vi "BRig_RT_panel_Laser1_v0,902.vi"(7 "input_setValues":bool, 9 "input_dataExp":u16[](array[numeric]), 11 "input_dataLC":u16[](array[numeric])) -> (1 "output_dataExp":u16[](array[numeric]), 3 "output_dataLC":u16[](array[numeric]))   [LabVIEW 2014]
panel:
  out "LaserPulseTrain":cluster{u16[], u16[]}(graph)
  in  "LED_baseline":bool
  in  "Laser_power_step":dbl
  in  "Laser_power_max":dbl
  in  "Laser_power_min":dbl
  in  "Laser_Tshutter":u16=2
  in  "Laser_Freq":u16=10
  in  "Laser_Tpeak":u16=2
  in  "Laser_T":u16
  in  "LC_Sel_PostR_Count":u16
  in  "LC_Sel_PostR_Probability":u16
  in  "LC_Sel_PostR_Block":u16(slide) max=2 step=1 scale=0.0..2.0
  in  "LC_Sel_PostR_OnOff":bool
  in  "LC_Sel_PostR_Tdelay":u16
  in  "LC_Cue_PostR_Count":u16
  in  "LC_Cue_PostR_delayOpt":bool
  in  "LC_Cue_PostR_Probability":u16
  in  "LC_Cue_PostR_Block":u16(slide) max=2 step=1 scale=0.0..2.0
  in  "LC_Cue_PostR_OnOff":bool
  in  "LC_Cue_PostR_Tdelay":u16
  in  "LC_ENL_PostR_delayOpt":bool
  in  "LC_ENL_PostR_Count":u16
  in  "LC_ENL_PostR_Probability":u16 max=100 step=1
  in  "LC_ENL_PostR_Block":u16(slide) max=2 step=1 scale=0.0..2.0
  in  "LC_ENL_PostR_OnOff":bool
  in  "LC_ENL_PostR_Tdelay":u16
  in  "LC_Sel_PreR_Count":u16
  in  "LC_Sel_First_Count":u16
  in  "LC_Sel_PreR_Probability":u16
  in  "LC_Sel_PreR_Block":u16(slide) max=2 step=1 scale=0.0..2.0
  in  "LC_Sel_PreR_OnOff":bool
  in  "LC_Sel_First_Probability":u16
  in  "LC_Sel_First_Block":u16(slide) max=2 step=1 scale=0.0..2.0
  in  "LC_Sel_First_OnOff":bool
  in  "LC_Sel_PreR_Tdelay":u16
  in  "LC_Sel_First_Tdelay":u16
  in  "LC_Cue_PreR_Count":u16
  in  "LC_Cue_First_Count":u16
  in  "LC_Cue_PreR_delayOpt":bool
  in  "LC_ENL_PreR_delayOpt":bool
  in  "LC_ENL_PreR_Count":u16
  in  "LC_ENL_First_Count":u16
  in  "LC_Cue_First_delayOpt":bool
  in  "LC_ENL_First_delayOpt":bool
  in  "LC_Wrong_Probability":u16
  in  "LC_Wrong_Trial":u16(slide) max=2 step=1 scale=0.0..2.0
  in  "LC_Wrong_Block":u16(slide) max=2 step=1 scale=0.0..2.0
  in  "LC_Wrong_OnOff":bool
  in  "LC_Reward_Probability":u16
  in  "LC_Reward_Trial":u16(slide) max=2 step=1 scale=0.0..2.0
  in  "LC_Reward_Block":u16(slide) max=2 step=1 scale=0.0..2.0
  in  "LC_Reward_OnOff":bool
  in  "LC_Cue_PreR_Probability":u16
  in  "LC_Cue_PreR_Block":u16(slide) max=2 step=1 scale=0.0..2.0
  in  "LC_Cue_PreR_OnOff":bool
  in  "LC_Cue_First_Probability":u16
  in  "LC_Cue_First_Block":u16(slide) max=2 step=1 scale=0.0..2.0
  in  "LC_Cue_First_OnOff":bool
  in  "LC_ENL_PreR_Probability":u16 max=100 step=1
  in  "LC_ENL_PreR_Block":u16(slide) max=2 step=1 scale=0.0..2.0
  in  "LC_ENL_PreR_OnOff":bool
  in  "LC_ENL_First_Probability":u16 max=100 step=1
  in  "LC_ENL_First_Block":u16(slide) max=2 step=1 scale=0.0..2.0
  in  "LC_Wrong_Tdelay":u16
  in  "LC_Cue_PreR_Tdelay":u16
  in  "LC_ENL_PreR_Tdelay":u16
  in  "LC_Reward_Tdelay":u16
  in  "LC_Cue_First_Tdelay":u16
  in  "LC_ENL_First_Tdelay":u16
  in  "LC_ENL_First_OnOff":bool
  # "Laser1 Control\n                               On/Off      Block        Probability [%]   Delay [ms]                              Count"
  # "Enforced\nNonLick"
  # "from end"
  # "First\nTrial"
  # "from start"
  # "from end"
  # "PreReward\nTrials"
  # "from start"
  # "from end"
  # "PostReward\nTrials"
  # "from start"
  # "Cue"
  # "from end"
  # "First\nTrial"
  # "from start"
  # "from end"
  # "PreReward\nTrials"
  # "from start"
  # "from end"
  # "PreReward\nTrials"
  # "from start"
  # "Selection"
  # "from start"
  # "First\nTrial"
  # "from start"
  # "PreReward\nTrials"
  # "from start"
  # "PostReward\nTrials"
  # "Laser1 Parameters"
  # "Laser1 Response\n           On/Off      Block           Trial     Probability %  Delay [ms]"
  # "Frequency\n[Hz]"
  # "Selection\nReward"
  # "Timing [ms]\n Duration     Peak Width   Shutter"
  # "Selection\nWrong"
  # "Laser Power [V]\nMin          Max              Step"
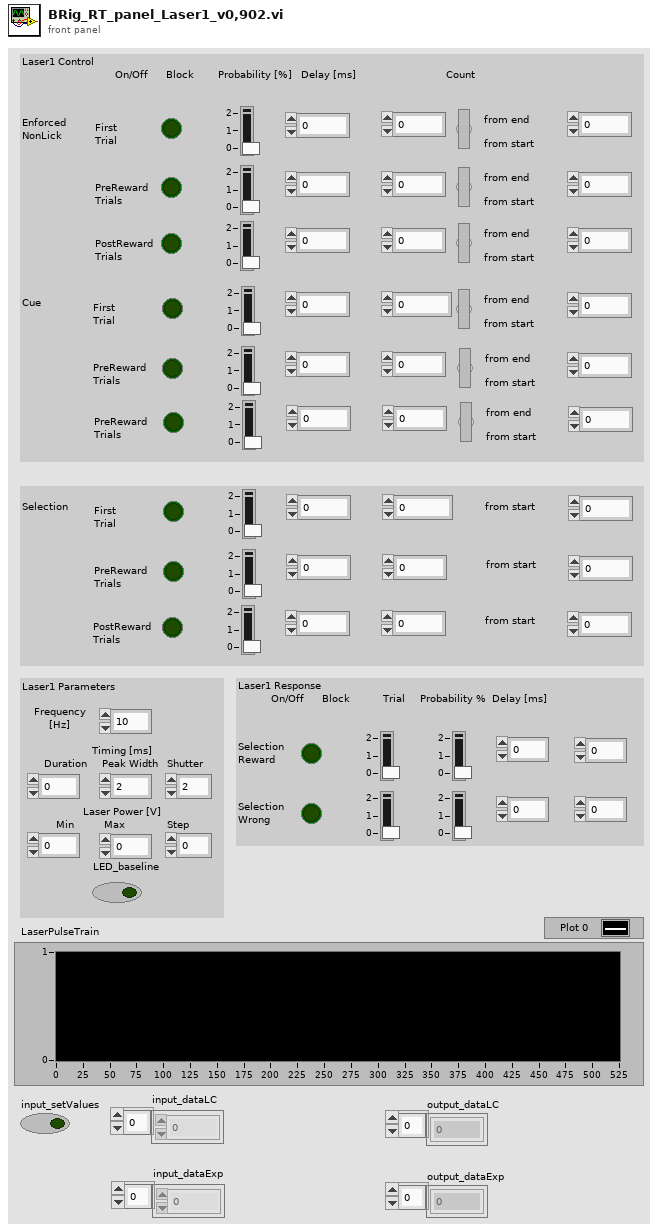
[diagram p1: front panel]
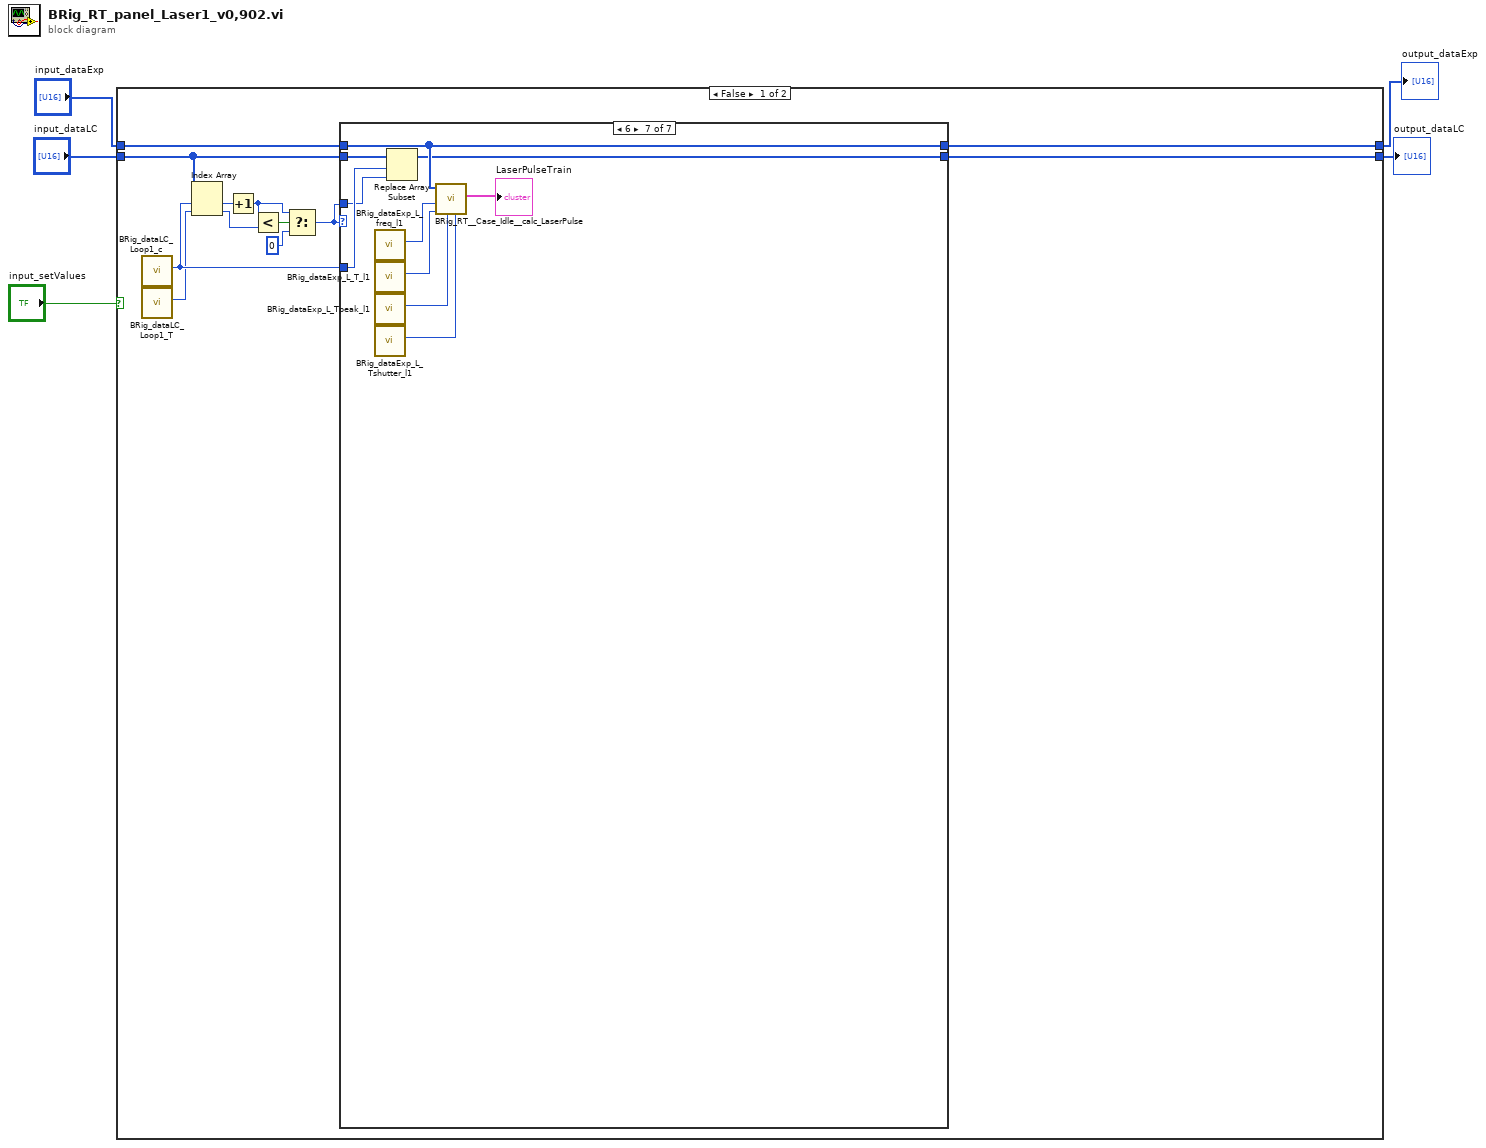
[diagram p0: block diagram]
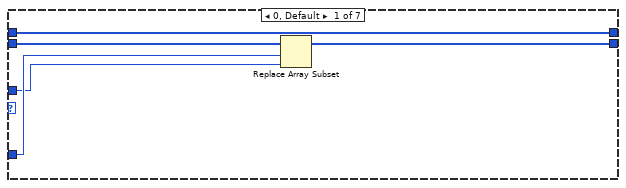
[diagram p2: hidden frame]
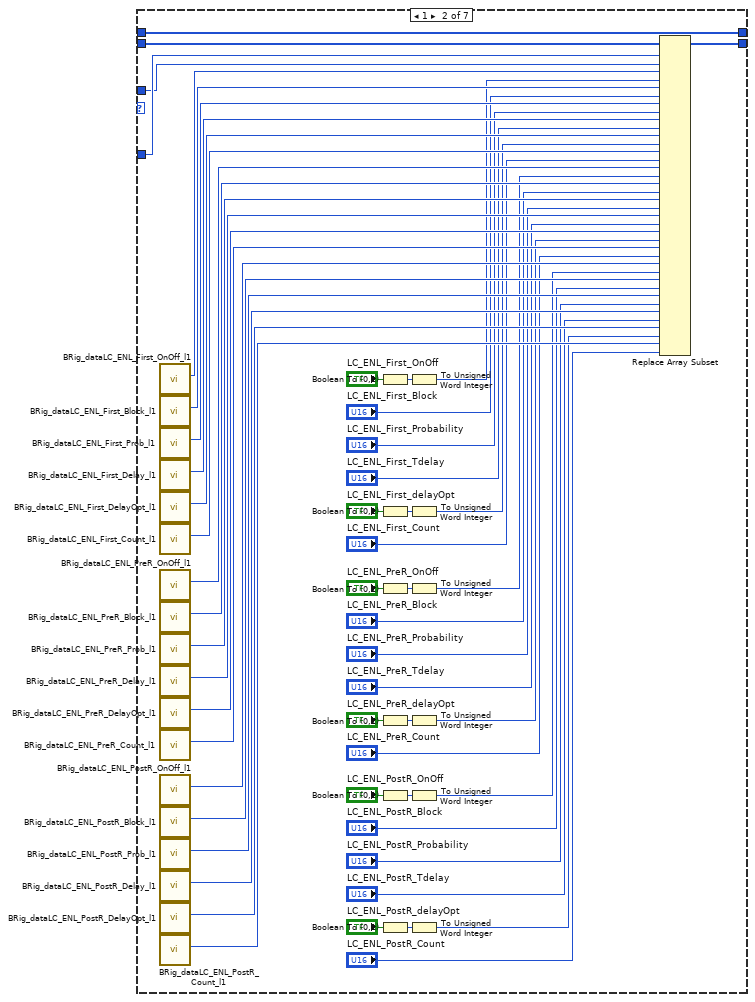
[diagram p3: hidden frame]
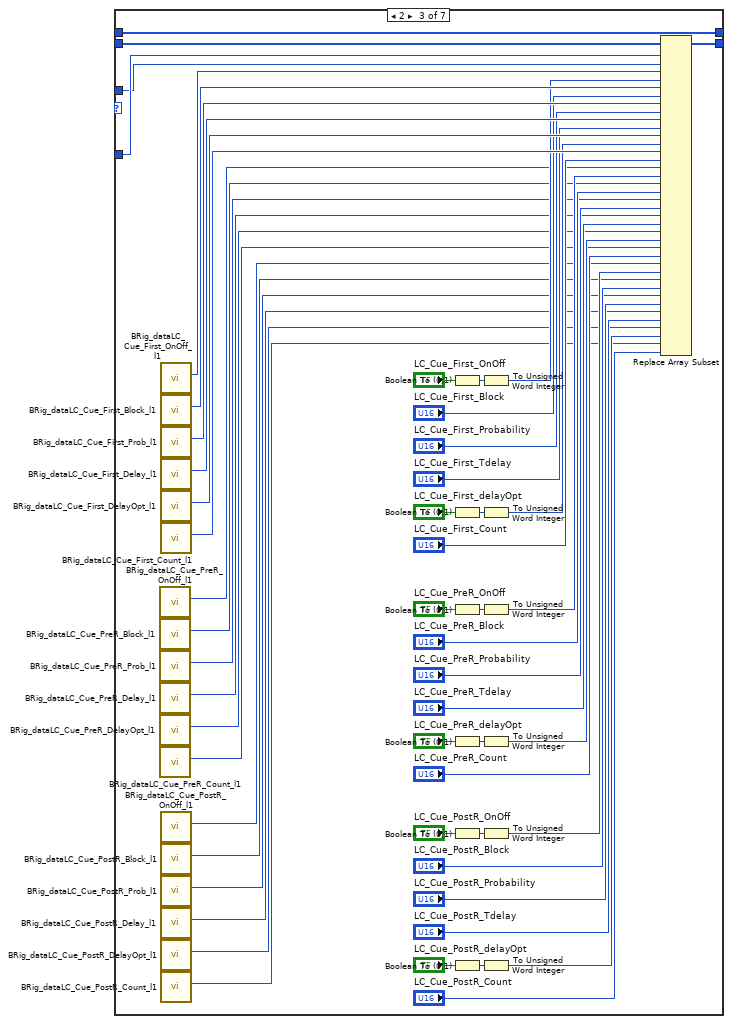
[diagram p4: hidden frame]
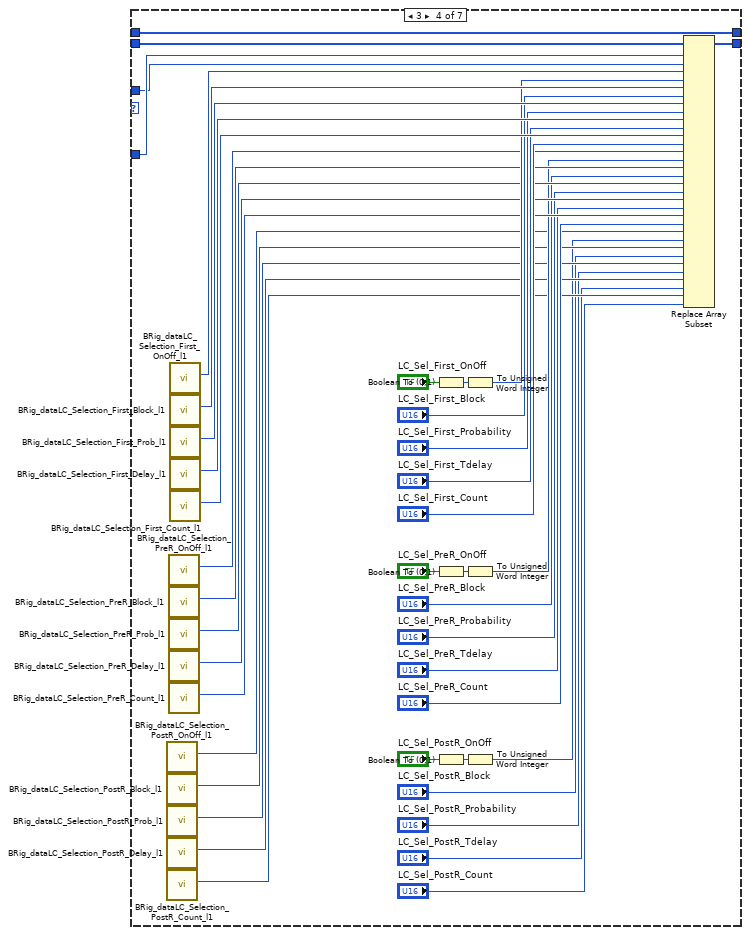
[diagram p5: hidden frame]
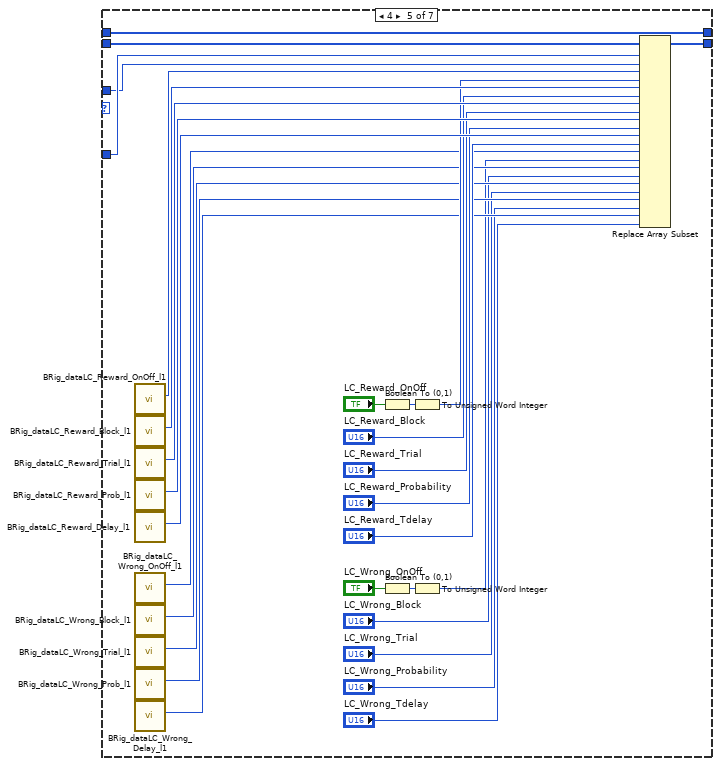
[diagram p6: hidden frame]
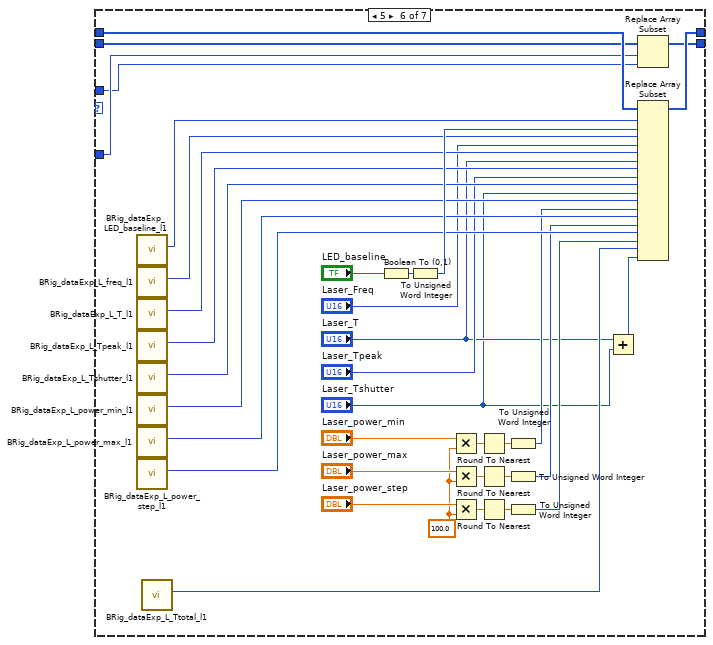
[diagram p7: hidden frame]
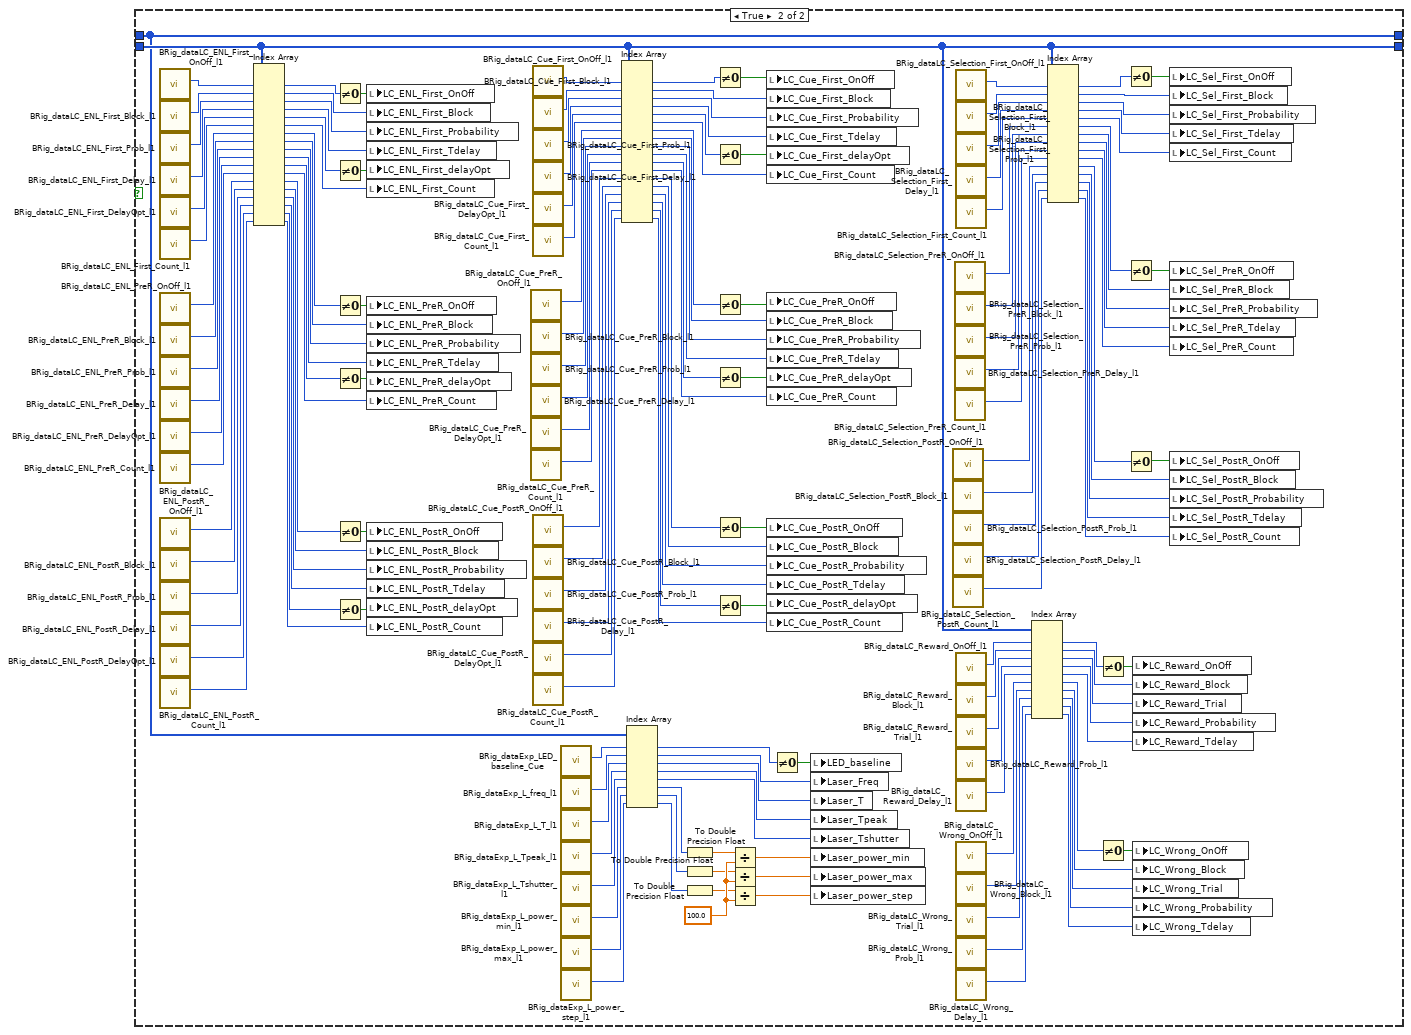
[diagram p8: hidden frame]
diagram:
  n1 = case shown="False" "input_setValues" {
    tunnel: "input_dataLC" -> [w17 w282]
    tunnel: [w11 w282] -> w4
    tunnel: "input_dataExp" -> [w7 w245]
    tunnel: [w6 w245] -> w1
    frame False {
      n2 = call "BRig_dataLC_Loop1_c.vi"() -> ("output_Loop1_c"=w10:i32)  [unwired: 11 in]
      n3 = call "BRig_dataLC_Loop1_T.vi"() -> ("output_Loop1_T"=w9:i32)  [unwired: 11 in]
      n4 = Index Array(array=w17, index #1=w10, index #2=w9) -> (element #1=w16:u16, element #2=w15:u16)
      n5 = Increment(x=w16) -> (x+1=w12:u16)
      n6 = Less?(x=w12, y=w15) -> (x < y?=w14:bool)
      n7 = Select(t=w12, s=w14, f=u16 0) -> (s? t:f=w8:u16)
      n8 = case shown="6" w8 {
        tunnel: w17 -> [w22 w75 w128 w169 w198 w203 w242]
        tunnel: w10 -> [w20 w25 w90 w131 w172 w201 w240]
        tunnel: w8 -> [w19 w24 w89 w130 w171 w200 w239]
        tunnel: [w21 w68 w127 w168 w197 w202 w241] -> w11
        tunnel: w7 -> [w18 w23 w76 w129 w170 w205 w244]
        tunnel: [w18 w23 w76 w129 w170 w204 w244] -> w6
        frame 0, Default {
          n9 = Replace Array Subset(array=w22, new element=w19, index=w20) -> (w21:u16[])
        }
        frame 1 {
          n10 = call "BRig_dataLC_ENL_First_OnOff_l1.vi"() -> ("output_ENL_First_OnOff"=w74:i32)  [unwired: 11 in]
          n11 = call "BRig_dataLC_ENL_First_Block_l1.vi"() -> ("output_ENL_First_Block"=w73:i32)  [unwired: 11 in]
          n12 = call "BRig_dataLC_ENL_First_Prob_l1.vi"() -> ("output_ENL_First_Prob"=w72:i32)  [unwired: 11 in]
          n13 = call "BRig_dataLC_ENL_First_Delay_l1.vi"() -> ("output_ENL_First_Delay"=w71:i32)  [unwired: 11 in]
          n14 = call "BRig_dataLC_ENL_First_DelayOpt_l1.vi"() -> ("output_ENL_First_DelayOpt"=w70:i32)  [unwired: 11 in]
          n15 = call "BRig_dataLC_ENL_First_Count_l1.vi"() -> ("output_ENL_First_Count"=w69:i32)  [unwired: 11 in]
          n16 = call "BRig_dataLC_ENL_PreR_OnOff_l1.vi"() -> ("output_ENL_PreR_OnOff"=w67:i32)  [unwired: 11 in]
          n17 = call "BRig_dataLC_ENL_PreR_Block_l1.vi"() -> ("output_ENL_PreR_Block"=w66:i32)  [unwired: 11 in]
          n18 = call "BRig_dataLC_ENL_PreR_Prob_l1.vi"() -> ("output_ENL_PreR_Prob"=w65:i32)  [unwired: 11 in]
          n19 = call "BRig_dataLC_ENL_PreR_Delay_l1.vi"() -> ("output_ENL_PreR_Delay"=w64:i32)  [unwired: 11 in]
          n20 = call "BRig_dataLC_ENL_PreR_DelayOpt_l1.vi"() -> ("output_ENL_PreR_DelayOpt"=w63:i32)  [unwired: 11 in]
          n21 = call "BRig_dataLC_ENL_PreR_Count_l1.vi"() -> ("output_ENL_PreR_Count"=w62:i32)  [unwired: 11 in]
          n22 = call "BRig_dataLC_ENL_PostR_OnOff_l1.vi"() -> ("output_ENL_PostR_OnOff"=w61:i32)  [unwired: 11 in]
          n23 = call "BRig_dataLC_ENL_PostR_Block_l1.vi"() -> ("output_ENL_PostR_Block"=w60:i32)  [unwired: 11 in]
          n24 = call "BRig_dataLC_ENL_PostR_Prob_l1.vi"() -> ("output_ENL_PostR_Prob"=w59:i32)  [unwired: 11 in]
          n25 = call "BRig_dataLC_ENL_PostR_Delay_l1.vi"() -> ("output_ENL_PostR_Delay"=w58:i32)  [unwired: 11 in]
          n26 = call "BRig_dataLC_ENL_PostR_DelayOpt_l1.vi"() -> ("output_ENL_PostR_DelayOpt"=w57:i32)  [unwired: 11 in]
          n27 = call "BRig_dataLC_ENL_PostR_Count_l1.vi"() -> ("output_ENL_PostR_Count"=w56:i32)  [unwired: 11 in]
          n28 = Boolean To (0,1)(Boolean="LC_ENL_First_OnOff") -> (0, 1=w54:i16)
          n29 = Boolean To (0,1)(Boolean="LC_ENL_First_delayOpt") -> (0, 1=w53:i16)
          n30 = Boolean To (0,1)(Boolean="LC_ENL_PreR_OnOff") -> (0, 1=w51:i16)
          n31 = Boolean To (0,1)(Boolean="LC_ENL_PreR_delayOpt") -> (0, 1=w49:i16)
          n32 = Boolean To (0,1)(Boolean="LC_ENL_PostR_OnOff") -> (0, 1=w47:i16)
          n33 = Boolean To (0,1)(Boolean="LC_ENL_PostR_delayOpt") -> (0, 1=w45:i16)
          n34 = To Unsigned Word Integer(number=w54) -> (unsigned 16bit integer=w43:u16)
          n35 = To Unsigned Word Integer(number=w53) -> (unsigned 16bit integer=w39:u16)
          n36 = To Unsigned Word Integer(number=w51) -> (unsigned 16bit integer=w37:u16)
          n37 = To Unsigned Word Integer(number=w49) -> (unsigned 16bit integer=w33:u16)
          n38 = To Unsigned Word Integer(number=w47) -> (unsigned 16bit integer=w31:u16)
          n39 = To Unsigned Word Integer(number=w45) -> (unsigned 16bit integer=w27:u16)
          n40 = Replace Array Subset(array=w75, new element #1=w24, index #1=w25, new element #2=w43, index #2=w74, new element #3="LC_ENL_First_Block", index #3=w73, new element #4="LC_ENL_First_Probability", index #4=w72, new element #5="LC_ENL_First_Tdelay", index #5=w71, new element #6=w39, index #6=w70, new element #7="LC_ENL_First_Count", index #7=w69, new element #8=w37, index #8=w67, new element #9="LC_ENL_PreR_Block", index #9=w66, new element #10="LC_ENL_PreR_Probability", index #10=w65, new element #11="LC_ENL_PreR_Tdelay", index #11=w64, new element #12=w33, index #12=w63, new element #13="LC_ENL_PreR_Count", index #13=w62, new element #14=w31, index #14=w61, new element #15="LC_ENL_PostR_Block", index #15=w60, new element #16="LC_ENL_PostR_Probability", index #16=w59, new element #17="LC_ENL_PostR_Tdelay", index #17=w58, new element #18=w27, index #18=w57, new element #19="LC_ENL_PostR_Count", index #19=w56) -> (w68:u16[])
        }
        frame 2 {
          n41 = call "BRig_dataLC_Cue_PreR_OnOff_l1.vi"() -> ("output_Cue_PreR_OnOff"=w86:i32)  [unwired: 11 in]
          n42 = call "BRig_dataLC_Cue_PreR_Block_l1.vi"() -> ("output_Cue_PreR_Block"=w85:i32)  [unwired: 11 in]
          n43 = call "BRig_dataLC_Cue_PreR_Prob_l1.vi"() -> ("output_Cue_PreR_Prob"=w84:i32)  [unwired: 11 in]
          n44 = call "BRig_dataLC_Cue_PreR_Delay_l1.vi"() -> ("output_Cue_PreR_Delay"=w83:i32)  [unwired: 11 in]
          n45 = call "BRig_dataLC_Cue_PreR_DelayOpt_l1.vi"() -> ("output_Cue_PreR_DelayOpt"=w82:i32)  [unwired: 11 in]
          n46 = call "BRig_dataLC_Cue_PreR_Count_l1.vi"() -> ("output_Cue_PreR_Count"=w87:i32)  [unwired: 11 in]
          n47 = call "BRig_dataLC_Cue_First_OnOff_l1.vi"() -> ("output_Cue_First_OnOff"=w126:i32)  [unwired: 11 in]
          n48 = call "BRig_dataLC_Cue_First_Block_l1.vi"() -> ("output_Cue_First_Block"=w125:i32)  [unwired: 11 in]
          n49 = call "BRig_dataLC_Cue_First_Prob_l1.vi"() -> ("output_Cue_First_Prob"=w124:i32)  [unwired: 11 in]
          n50 = call "BRig_dataLC_Cue_First_Delay_l1.vi"() -> ("output_Cue_First_Delay"=w123:i32)  [unwired: 11 in]
          n51 = call "BRig_dataLC_Cue_First_DelayOpt_l1.vi"() -> ("output_Cue_First_DelayOpt"=w122:i32)  [unwired: 11 in]
          n52 = call "BRig_dataLC_Cue_First_Count_l1.vi"() -> ("output_Cue_First_Count"=w121:i32)  [unwired: 11 in]
          n53 = call "BRig_dataLC_Cue_PostR_OnOff_l1.vi"() -> ("output_Cue_PostR_OnOff"=w88:i32)  [unwired: 11 in]
          n54 = call "BRig_dataLC_Cue_PostR_Block_l1.vi"() -> ("output_Cue_PostR_Block"=w81:i32)  [unwired: 11 in]
          n55 = call "BRig_dataLC_Cue_PostR_Prob_l1.vi"() -> ("output_Cue_PostR_Prob"=w80:i32)  [unwired: 11 in]
          n56 = call "BRig_dataLC_Cue_PostR_Delay_l1.vi"() -> ("output_Cue_PostR_Delay"=w79:i32)  [unwired: 11 in]
          n57 = call "BRig_dataLC_Cue_PostR_DelayOpt_l1.vi"() -> ("output_Cue_PostR_DelayOpt"=w78:i32)  [unwired: 11 in]
          n58 = call "BRig_dataLC_Cue_PostR_Count_l1.vi"() -> ("output_Cue_PostR_Count"=w77:i32)  [unwired: 11 in]
          n59 = Boolean To (0,1)(Boolean="LC_Cue_First_OnOff") -> (0, 1=w114:i16)
          n60 = Boolean To (0,1)(Boolean="LC_Cue_First_delayOpt") -> (0, 1=w113:i16)
          n61 = Boolean To (0,1)(Boolean="LC_Cue_PreR_OnOff") -> (0, 1=w112:i16)
          n62 = Boolean To (0,1)(Boolean="LC_Cue_PreR_delayOpt") -> (0, 1=w111:i16)
          n63 = Boolean To (0,1)(Boolean="LC_Cue_PostR_OnOff") -> (0, 1=w110:i16)
          n64 = Boolean To (0,1)(Boolean="LC_Cue_PostR_delayOpt") -> (0, 1=w109:i16)
          n65 = To Unsigned Word Integer(number=w114) -> (unsigned 16bit integer=w108:u16)
          n66 = To Unsigned Word Integer(number=w113) -> (unsigned 16bit integer=w104:u16)
          n67 = To Unsigned Word Integer(number=w112) -> (unsigned 16bit integer=w102:u16)
          n68 = To Unsigned Word Integer(number=w111) -> (unsigned 16bit integer=w98:u16)
          n69 = To Unsigned Word Integer(number=w110) -> (unsigned 16bit integer=w96:u16)
          n70 = To Unsigned Word Integer(number=w109) -> (unsigned 16bit integer=w92:u16)
          n71 = Replace Array Subset(array=w128, new element #1=w89, index #1=w90, new element #2=w108, index #2=w126, new element #3="LC_Cue_First_Block", index #3=w125, new element #4="LC_Cue_First_Probability", index #4=w124, new element #5="LC_Cue_First_Tdelay", index #5=w123, new element #6=w104, index #6=w122, new element #7="LC_Cue_First_Count", index #7=w121, new element #8=w102, index #8=w86, new element #9="LC_Cue_PreR_Block", index #9=w85, new element #10="LC_Cue_PreR_Probability", index #10=w84, new element #11="LC_Cue_PreR_Tdelay", index #11=w83, new element #12=w98, index #12=w82, new element #13="LC_Cue_PreR_Count", index #13=w87, new element #14=w96, index #14=w88, new element #15="LC_Cue_PostR_Block", index #15=w81, new element #16="LC_Cue_PostR_Probability", index #16=w80, new element #17="LC_Cue_PostR_Tdelay", index #17=w79, new element #18=w92, index #18=w78, new element #19="LC_Cue_PostR_Count", index #19=w77) -> (w127:u16[])
        }
        frame 3 {
          n72 = call "BRig_dataLC_Selection_PostR_OnOff_l1.vi"() -> ("output_Selection_PostR_OnOff"=w141:i32)  [unwired: 11 in]
          n73 = call "BRig_dataLC_Selection_PostR_Block_l1.vi"() -> ("output_Selection_PostR_Block"=w140:i32)  [unwired: 11 in]
          n74 = call "BRig_dataLC_Selection_PostR_Prob_l1.vi"() -> ("output_Selection_PostR_Prob"=w139:i32)  [unwired: 11 in]
          n75 = call "BRig_dataLC_Selection_PostR_Delay_l1.vi"() -> ("output_Selection_PostR_Delay"=w138:i32)  [unwired: 11 in]
          n76 = call "BRig_dataLC_Selection_PostR_Count_l1.vi"() -> ("output_Selection_PostR_Count"=w137:i32)  [unwired: 11 in]
          n77 = call "BRig_dataLC_Selection_PreR_OnOff_l1.vi"() -> ("output_Selection_PreR_OnOff"=w151:i32)  [unwired: 11 in]
          n78 = call "BRig_dataLC_Selection_PreR_Block_l1.vi"() -> ("output_Selection_PreR_Block"=w150:i32)  [unwired: 11 in]
          n79 = call "BRig_dataLC_Selection_PreR_Prob_l1.vi"() -> ("output_Selection_PreR_Prob"=w149:i32)  [unwired: 11 in]
          n80 = call "BRig_dataLC_Selection_PreR_Delay_l1.vi"() -> ("output_Selection_PreR_Delay"=w148:i32)  [unwired: 11 in]
          n81 = call "BRig_dataLC_Selection_PreR_Count_l1.vi"() -> ("output_Selection_PreR_Count"=w147:i32)  [unwired: 11 in]
          n82 = call "BRig_dataLC_Selection_First_OnOff_l1.vi"() -> ("output_Selection_First_OnOff"=w161:i32)  [unwired: 11 in]
          n83 = call "BRig_dataLC_Selection_First_Block_l1.vi"() -> ("output_Selection_First_Block"=w160:i32)  [unwired: 11 in]
          n84 = call "BRig_dataLC_Selection_First_Prob_l1.vi"() -> ("output_Selection_First_Prob"=w159:i32)  [unwired: 11 in]
          n85 = call "BRig_dataLC_Selection_First_Delay_l1.vi"() -> ("output_Selection_First_Delay"=w158:i32)  [unwired: 11 in]
          n86 = call "BRig_dataLC_Selection_First_Count_l1.vi"() -> ("output_Selection_First_Count"=w157:i32)  [unwired: 11 in]
          n87 = Boolean To (0,1)(Boolean="LC_Sel_First_OnOff") -> (0, 1=w164:i16)
          n88 = Boolean To (0,1)(Boolean="LC_Sel_PreR_OnOff") -> (0, 1=w163:i16)
          n89 = Boolean To (0,1)(Boolean="LC_Sel_PostR_OnOff") -> (0, 1=w162:i16)
          n90 = To Unsigned Word Integer(number=w164) -> (unsigned 16bit integer=w156:u16)
          n91 = To Unsigned Word Integer(number=w163) -> (unsigned 16bit integer=w146:u16)
          n92 = To Unsigned Word Integer(number=w162) -> (unsigned 16bit integer=w136:u16)
          n93 = Replace Array Subset(array=w169, new element #1=w130, index #1=w131, new element #2=w156, index #2=w161, new element #3="LC_Sel_First_Block", index #3=w160, new element #4="LC_Sel_First_Probability", index #4=w159, new element #5="LC_Sel_First_Tdelay", index #5=w158, new element #6="LC_Sel_First_Count", index #6=w157, new element #7=w146, index #7=w151, new element #8="LC_Sel_PreR_Block", index #8=w150, new element #9="LC_Sel_PreR_Probability", index #9=w149, new element #10="LC_Sel_PreR_Tdelay", index #10=w148, new element #11="LC_Sel_PreR_Count", index #11=w147, new element #12=w136, index #12=w141, new element #13="LC_Sel_PostR_Block", index #13=w140, new element #14="LC_Sel_PostR_Probability", index #14=w139, new element #15="LC_Sel_PostR_Tdelay", index #15=w138, new element #16="LC_Sel_PostR_Count", index #16=w137) -> (w168:u16[])
        }
        frame 4 {
          n94 = call "BRig_dataLC_Reward_OnOff_l1.vi"() -> ("output_Reward_OnOff"=w196:i32)  [unwired: 11 in]
          n95 = call "BRig_dataLC_Reward_Block_l1.vi"() -> ("output_Reward_Block"=w195:i32)  [unwired: 11 in]
          n96 = call "BRig_dataLC_Reward_Trial_l1.vi"() -> ("output_Reward_Trial"=w194:i32)  [unwired: 11 in]
          n97 = call "BRig_dataLC_Reward_Prob_l1.vi"() -> ("output_Reward_Prob"=w193:i32)  [unwired: 11 in]
          n98 = call "BRig_dataLC_Reward_Delay_l1.vi"() -> ("output_Reward_Delay"=w192:i32)  [unwired: 11 in]
          n99 = call "BRig_dataLC_Wrong_OnOff_l1.vi"() -> ("output_Wrong_OnOff"=w182:i32)  [unwired: 11 in]
          n100 = call "BRig_dataLC_Wrong_Block_l1.vi"() -> ("output_Wrong_Block"=w181:i32)  [unwired: 11 in]
          n101 = call "BRig_dataLC_Wrong_Trial_l1.vi"() -> ("output_Wrong_Trial"=w180:i32)  [unwired: 11 in]
          n102 = call "BRig_dataLC_Wrong_Prob_l1.vi"() -> ("output_Wrong_Prob"=w179:i32)  [unwired: 11 in]
          n103 = call "BRig_dataLC_Wrong_Delay_l1.vi"() -> ("output_Wrong_Delay"=w178:i32)  [unwired: 11 in]
          n104 = Boolean To (0,1)(Boolean="LC_Reward_OnOff") -> (0, 1=w189:i16)
          n105 = Boolean To (0,1)(Boolean="LC_Wrong_OnOff") -> (0, 1=w188:i16)
          n106 = To Unsigned Word Integer(number=w189) -> (unsigned 16bit integer=w187:u16)
          n107 = To Unsigned Word Integer(number=w188) -> (unsigned 16bit integer=w177:u16)
          n108 = Replace Array Subset(array=w198, new element #1=w171, index #1=w172, new element #2=w187, index #2=w196, new element #3="LC_Reward_Block", index #3=w195, new element #4="LC_Reward_Trial", index #4=w194, new element #5="LC_Reward_Probability", index #5=w193, new element #6="LC_Reward_Tdelay", index #6=w192, new element #7=w177, index #7=w182, new element #8="LC_Wrong_Block", index #8=w181, new element #9="LC_Wrong_Trial", index #9=w180, new element #10="LC_Wrong_Probability", index #10=w179, new element #11="LC_Wrong_Tdelay", index #11=w178) -> (w197:u16[])
        }
        frame 5 {
          w222 = 100.0 ("y")
          n109 = call "BRig_dataExp_LED_baseline_l1.vi"() -> ("output_LED_baseline_l1"=w199:i32)  [unwired: 11 in]
          n110 = call "BRig_dataExp_L_freq_l1.vi"() -> ("output_L_freq_l1"=w221:i32)  [unwired: 11 in]
          n111 = call "BRig_dataExp_L_T_l1.vi"() -> ("output_L_T_l1"=w220:i32)  [unwired: 11 in]
          n112 = call "BRig_dataExp_L_Tpeak_l1.vi"() -> ("output_L_Tpeak_l1"=w219:i32)  [unwired: 11 in]
          n113 = call "BRig_dataExp_L_Tshutter_l1.vi"() -> ("output_L_Tshutter_l1"=w218:i32)  [unwired: 11 in]
          n114 = call "BRig_dataExp_L_power_min_l1.vi"() -> ("output_L_power_min_l1"=w217:i32)  [unwired: 11 in]
          n115 = call "BRig_dataExp_L_power_max_l1.vi"() -> ("output_L_power_max_l1"=w216:i32)  [unwired: 11 in]
          n116 = call "BRig_dataExp_L_power_step_l1.vi"() -> ("output_L_power_step_l1"=w215:i32)  [unwired: 11 in]
          n117 = call "BRig_dataExp_L_Ttotal_l1.vi"() -> ("output_L_Ttotal_l1"=w209:i32)  [unwired: 11 in]
          n118 = Boolean To (0,1)(Boolean="LED_baseline") -> (0, 1=w234:i16)
          n119 = To Unsigned Word Integer(number=w234) -> (unsigned 16bit integer=w232:u16)
          n120 = Multiply(x="Laser_power_min", y=w222) -> (x*y=w226:dbl)
          n121 = Multiply(x="Laser_power_max", y=w222) -> (x*y=w228:dbl)
          n122 = Multiply(x="Laser_power_step", y=w222) -> (x*y=w231:dbl)
          n123 = Round To Nearest(number=w226) -> (nearest integer value=w225:dbl)
          n124 = Round To Nearest(number=w228) -> (nearest integer value=w227:dbl)
          n125 = Round To Nearest(number=w231) -> (nearest integer value=w230:dbl)
          n126 = To Unsigned Word Integer(number=w225) -> (unsigned 16bit integer=w212:u16)
          n127 = To Unsigned Word Integer(number=w227) -> (unsigned 16bit integer=w213:u16)
          n128 = To Unsigned Word Integer(number=w230) -> (unsigned 16bit integer=w214:u16)
          n129 = Add(x="Laser_T", y="Laser_Tshutter") -> (x+y=w206:u16)
          n130 = Replace Array Subset(array=w203, new element=w200, index=w201) -> (w202:u16[])
          n131 = Replace Array Subset(array=w205, new element #1=w232, index #1=w199, new element #2="Laser_Freq", index #2=w221, new element #3="Laser_T", index #3=w220, new element #4="Laser_Tpeak", index #4=w219, new element #5="Laser_Tshutter", index #5=w218, new element #6=w212, index #6=w217, new element #7=w213, index #7=w216, new element #8=w214, index #8=w215, new element #9=w206, index #9=w209) -> (w204:u16[])
        }
        frame 6 {
          n132 = call "BRig_dataExp_L_freq_l1.vi"() -> ("output_L_freq_l1"=w237:i32)  [unwired: 11 in]
          n133 = call "BRig_dataExp_L_T_l1.vi"() -> ("output_L_T_l1"=w238:i32)  [unwired: 11 in]
          n134 = call "BRig_dataExp_L_Tpeak_l1.vi"() -> ("output_L_Tpeak_l1"=w236:i32)  [unwired: 11 in]
          n135 = call "BRig_dataExp_L_Tshutter_l1.vi"() -> ("output_L_Tshutter_l1"=w235:i32)  [unwired: 11 in]
          n136 = Replace Array Subset(array=w242, new element=w239, index=w240) -> (w241:u16[])
          n137 = call "BRig_RT__Case_Idle__calc_LaserPulse.vi"("input_dataExp_L_Tshutter"=w235, "input_dataExp_L_Tpeak"=w236, "input_dataExp_L_T"=w238, "input_dataExp_L_freq"=w237, "input_dataExp"=w244) -> ("output_cluster"=→"LaserPulseTrain":cluster{u16[], u16[]})  [unwired: 6 in]
        }
      }
    }
    frame True {
      w260 = 100.0 ("y")
      n138 = call "BRig_dataLC_ENL_First_OnOff_l1.vi"() -> ("output_ENL_First_OnOff"=w403:i32)  [unwired: 11 in]
      n139 = call "BRig_dataLC_ENL_First_Block_l1.vi"() -> ("output_ENL_First_Block"=w402:i32)  [unwired: 11 in]
      n140 = call "BRig_dataLC_ENL_First_Prob_l1.vi"() -> ("output_ENL_First_Prob"=w401:i32)  [unwired: 11 in]
      n141 = call "BRig_dataLC_ENL_First_Delay_l1.vi"() -> ("output_ENL_First_Delay"=w400:i32)  [unwired: 11 in]
      n142 = call "BRig_dataLC_ENL_First_DelayOpt_l1.vi"() -> ("output_ENL_First_DelayOpt"=w399:i32)  [unwired: 11 in]
      n143 = call "BRig_dataLC_ENL_First_Count_l1.vi"() -> ("output_ENL_First_Count"=w398:i32)  [unwired: 11 in]
      n144 = call "BRig_dataLC_ENL_PreR_OnOff_l1.vi"() -> ("output_ENL_PreR_OnOff"=w397:i32)  [unwired: 11 in]
      n145 = call "BRig_dataLC_ENL_PreR_Block_l1.vi"() -> ("output_ENL_PreR_Block"=w396:i32)  [unwired: 11 in]
      n146 = call "BRig_dataLC_ENL_PreR_Prob_l1.vi"() -> ("output_ENL_PreR_Prob"=w395:i32)  [unwired: 11 in]
      n147 = call "BRig_dataLC_ENL_PreR_Delay_l1.vi"() -> ("output_ENL_PreR_Delay"=w394:i32)  [unwired: 11 in]
      n148 = call "BRig_dataLC_ENL_PreR_DelayOpt_l1.vi"() -> ("output_ENL_PreR_DelayOpt"=w393:i32)  [unwired: 11 in]
      n149 = call "BRig_dataLC_ENL_PreR_Count_l1.vi"() -> ("output_ENL_PreR_Count"=w392:i32)  [unwired: 11 in]
      n150 = call "BRig_dataLC_ENL_PostR_OnOff_l1.vi"() -> ("output_ENL_PostR_OnOff"=w391:i32)  [unwired: 11 in]
      n151 = call "BRig_dataLC_ENL_PostR_Block_l1.vi"() -> ("output_ENL_PostR_Block"=w390:i32)  [unwired: 11 in]
      n152 = call "BRig_dataLC_ENL_PostR_Prob_l1.vi"() -> ("output_ENL_PostR_Prob"=w389:i32)  [unwired: 11 in]
      n153 = call "BRig_dataLC_ENL_PostR_Delay_l1.vi"() -> ("output_ENL_PostR_Delay"=w388:i32)  [unwired: 11 in]
      n154 = call "BRig_dataLC_ENL_PostR_DelayOpt_l1.vi"() -> ("output_ENL_PostR_DelayOpt"=w387:i32)  [unwired: 11 in]
      n155 = call "BRig_dataLC_ENL_PostR_Count_l1.vi"() -> ("output_ENL_PostR_Count"=w386:i32)  [unwired: 11 in]
      n156 = Index Array(array=w282, index #1=w403, index #2=w402, index #3=w401, index #4=w400, index #5=w399, index #6=w398, index #7=w397, index #8=w396, index #9=w395, index #10=w394, index #11=w393, index #12=w392, index #13=w391, index #14=w390, index #15=w389, index #16=w388, index #17=w387, index #18=w386) -> (element #1=w379:u16, element #2=w378:u16, element #3=w377:u16, element #4=w376:u16, element #5=w375:u16, element #6=w374:u16, element #7=w373:u16, element #8=w372:u16, element #9=w371:u16, element #10=w370:u16, element #11=w369:u16, element #12=w368:u16, element #13=w367:u16, element #14=w366:u16, element #15=w365:u16, element #16=w364:u16, element #17=w363:u16, element #18=w362:u16)
      n157 = Not Equal To 0?(x=w379) -> (x != 0?=w385:bool)
      n158 = Not Equal To 0?(x=w375) -> (x != 0?=w384:bool)
      n159 = Not Equal To 0?(x=w373) -> (x != 0?=w383:bool)
      n160 = Not Equal To 0?(x=w369) -> (x != 0?=w382:bool)
      n161 = Not Equal To 0?(x=w367) -> (x != 0?=w381:bool)
      n162 = Not Equal To 0?(x=w363) -> (x != 0?=w380:bool)
      n163 = local write "LC_ENL_First_OnOff"(w385) -> ()
      n164 = local write "LC_ENL_First_Block"(w378) -> ()
      n165 = local write "LC_ENL_First_Probability"(w377) -> ()
      n166 = local write "LC_ENL_First_Tdelay"(w376) -> ()
      n167 = local write "LC_ENL_First_delayOpt"(w384) -> ()
      n168 = local write "LC_ENL_First_Count"(w374) -> ()
      n169 = local write "LC_ENL_PreR_OnOff"(w383) -> ()
      n170 = local write "LC_ENL_PreR_Block"(w372) -> ()
      n171 = local write "LC_ENL_PreR_Probability"(w371) -> ()
      n172 = local write "LC_ENL_PreR_Tdelay"(w370) -> ()
      n173 = local write "LC_ENL_PreR_delayOpt"(w382) -> ()
      n174 = local write "LC_ENL_PreR_Count"(w368) -> ()
      n175 = local write "LC_ENL_PostR_OnOff"(w381) -> ()
      n176 = local write "LC_ENL_PostR_Block"(w366) -> ()
      n177 = local write "LC_ENL_PostR_Probability"(w365) -> ()
      n178 = local write "LC_ENL_PostR_Tdelay"(w364) -> ()
      n179 = local write "LC_ENL_PostR_delayOpt"(w380) -> ()
      n180 = local write "LC_ENL_PostR_Count"(w362) -> ()
      n181 = call "BRig_dataLC_Cue_PreR_OnOff_l1.vi"() -> ("output_Cue_PreR_OnOff"=w250:i32)  [unwired: 11 in]
      n182 = call "BRig_dataLC_Cue_PreR_Block_l1.vi"() -> ("output_Cue_PreR_Block"=w249:i32)  [unwired: 11 in]
      n183 = call "BRig_dataLC_Cue_PreR_Prob_l1.vi"() -> ("output_Cue_PreR_Prob"=w248:i32)  [unwired: 11 in]
      n184 = call "BRig_dataLC_Cue_PreR_Delay_l1.vi"() -> ("output_Cue_PreR_Delay"=w247:i32)  [unwired: 11 in]
      n185 = call "BRig_dataLC_Cue_PreR_DelayOpt_l1.vi"() -> ("output_Cue_PreR_DelayOpt"=w246:i32)  [unwired: 11 in]
      n186 = call "BRig_dataLC_Cue_PreR_Count_l1.vi"() -> ("output_Cue_PreR_Count"=w251:i32)  [unwired: 11 in]
      n187 = call "BRig_dataLC_Cue_First_OnOff_l1.vi"() -> ("output_Cue_First_OnOff"=w409:i32)  [unwired: 11 in]
      n188 = call "BRig_dataLC_Cue_First_Block_l1.vi"() -> ("output_Cue_First_Block"=w408:i32)  [unwired: 11 in]
      n189 = call "BRig_dataLC_Cue_First_Prob_l1.vi"() -> ("output_Cue_First_Prob"=w407:i32)  [unwired: 11 in]
      n190 = call "BRig_dataLC_Cue_First_Delay_l1.vi"() -> ("output_Cue_First_Delay"=w406:i32)  [unwired: 11 in]
      n191 = call "BRig_dataLC_Cue_First_DelayOpt_l1.vi"() -> ("output_Cue_First_DelayOpt"=w405:i32)  [unwired: 11 in]
      n192 = call "BRig_dataLC_Cue_First_Count_l1.vi"() -> ("output_Cue_First_Count"=w404:i32)  [unwired: 11 in]
      n193 = call "BRig_dataLC_Cue_PostR_OnOff_l1.vi"() -> ("output_Cue_PostR_OnOff"=w256:i32)  [unwired: 11 in]
      n194 = call "BRig_dataLC_Cue_PostR_Block_l1.vi"() -> ("output_Cue_PostR_Block"=w255:i32)  [unwired: 11 in]
      n195 = call "BRig_dataLC_Cue_PostR_Prob_l1.vi"() -> ("output_Cue_PostR_Prob"=w254:i32)  [unwired: 11 in]
      n196 = call "BRig_dataLC_Cue_PostR_Delay_l1.vi"() -> ("output_Cue_PostR_Delay"=w253:i32)  [unwired: 11 in]
      n197 = call "BRig_dataLC_Cue_PostR_DelayOpt_l1.vi"() -> ("output_Cue_PostR_DelayOpt"=w252:i32)  [unwired: 11 in]
      n198 = call "BRig_dataLC_Cue_PostR_Count_l1.vi"() -> ("output_Cue_PostR_Count"=w257:i32)  [unwired: 11 in]
      n199 = call "BRig_dataExp_LED_baseline_Cue.vi"() -> ("output_LED_baseline_Cue"=w281:i32)  [unwired: 11 in]
      n200 = call "BRig_dataExp_L_freq_l1.vi"() -> ("output_L_freq_l1"=w280:i32)  [unwired: 11 in]
      n201 = call "BRig_dataExp_L_T_l1.vi"() -> ("output_L_T_l1"=w279:i32)  [unwired: 11 in]
      n202 = call "BRig_dataExp_L_Tpeak_l1.vi"() -> ("output_L_Tpeak_l1"=w278:i32)  [unwired: 11 in]
      n203 = call "BRig_dataExp_L_Tshutter_l1.vi"() -> ("output_L_Tshutter_l1"=w277:i32)  [unwired: 11 in]
      n204 = call "BRig_dataExp_L_power_min_l1.vi"() -> ("output_L_power_min_l1"=w276:i32)  [unwired: 11 in]
      n205 = call "BRig_dataExp_L_power_max_l1.vi"() -> ("output_L_power_max_l1"=w275:i32)  [unwired: 11 in]
      n206 = call "BRig_dataExp_L_power_step_l1.vi"() -> ("output_L_power_step_l1"=w274:i32)  [unwired: 11 in]
      n207 = Index Array(array=w282, index #1=w409, index #2=w408, index #3=w407, index #4=w406, index #5=w405, index #6=w404, index #7=w250, index #8=w249, index #9=w248, index #10=w247, index #11=w246, index #12=w251, index #13=w256, index #14=w255, index #15=w254, index #16=w253, index #17=w252, index #18=w257) -> (element #1=w355:u16, element #2=w354:u16, element #3=w353:u16, element #4=w352:u16, element #5=w351:u16, element #6=w350:u16, element #7=w349:u16, element #8=w348:u16, element #9=w347:u16, element #10=w346:u16, element #11=w345:u16, element #12=w344:u16, element #13=w343:u16, element #14=w342:u16, element #15=w341:u16, element #16=w340:u16, element #17=w339:u16, element #18=w338:u16)
      n208 = Index Array(array=w245, index #1=w281, index #2=w280, index #3=w279, index #4=w278, index #5=w277, index #6=w276, index #7=w275, index #8=w274) -> (element #1=w273:u16, element #2=w271:u16, element #3=w270:u16, element #4=w269:u16, element #5=w268:u16, element #6=w267:u16, element #7=w266:u16, element #8=w265:u16)
      n209 = To Double Precision Float(number=w267) -> (double precision float=w264:dbl)
      n210 = To Double Precision Float(number=w266) -> (double precision float=w259:dbl)
      n211 = To Double Precision Float(number=w265) -> (double precision float=w258:dbl)
      n212 = Not Equal To 0?(x=w355) -> (x != 0?=w361:bool)
      n213 = Not Equal To 0?(x=w351) -> (x != 0?=w360:bool)
      n214 = Not Equal To 0?(x=w349) -> (x != 0?=w359:bool)
      n215 = Not Equal To 0?(x=w345) -> (x != 0?=w358:bool)
      n216 = Not Equal To 0?(x=w343) -> (x != 0?=w357:bool)
      n217 = Not Equal To 0?(x=w339) -> (x != 0?=w356:bool)
      n218 = Divide(x=w264, y=w260) -> (x/y=w263:dbl)
      n219 = Divide(x=w259, y=w260) -> (x/y=w262:dbl)
      n220 = Divide(x=w258, y=w260) -> (x/y=w261:dbl)
      n221 = local write "LC_Cue_First_OnOff"(w361) -> ()
      n222 = local write "LC_Cue_First_Block"(w354) -> ()
      n223 = local write "LC_Cue_First_Probability"(w353) -> ()
      n224 = local write "LC_Cue_First_Tdelay"(w352) -> ()
      n225 = local write "LC_Cue_First_delayOpt"(w360) -> ()
      n226 = local write "LC_Cue_First_Count"(w350) -> ()
      n227 = local write "LC_Cue_PreR_OnOff"(w359) -> ()
      n228 = local write "LC_Cue_PreR_Block"(w348) -> ()
      n229 = local write "LC_Cue_PreR_Probability"(w347) -> ()
      n230 = local write "LC_Cue_PreR_Tdelay"(w346) -> ()
      n231 = local write "LC_Cue_PreR_delayOpt"(w358) -> ()
      n232 = local write "LC_Cue_PreR_Count"(w344) -> ()
      n233 = local write "LC_Cue_PostR_OnOff"(w357) -> ()
      n234 = local write "LC_Cue_PostR_Block"(w342) -> ()
      n235 = local write "LC_Cue_PostR_Probability"(w341) -> ()
      n236 = local write "LC_Cue_PostR_Tdelay"(w340) -> ()
      n237 = local write "LC_Cue_PostR_delayOpt"(w356) -> ()
      n238 = local write "LC_Cue_PostR_Count"(w338) -> ()
      n239 = Not Equal To 0?(x=w273) -> (x != 0?=w272:bool)
      n240 = local write "LED_baseline"(w272) -> ()
      n241 = local write "Laser_Freq"(w271) -> ()
      n242 = local write "Laser_T"(w270) -> ()
      n243 = local write "Laser_Tpeak"(w269) -> ()
      n244 = local write "Laser_Tshutter"(w268) -> ()
      n245 = local write "Laser_power_min"(w263) -> ()
      n246 = local write "Laser_power_max"(w262) -> ()
      n247 = local write "Laser_power_step"(w261) -> ()
      n248 = call "BRig_dataLC_Selection_PostR_OnOff_l1.vi"() -> ("output_Selection_PostR_OnOff"=w327:i32)  [unwired: 11 in]
      n249 = call "BRig_dataLC_Selection_PostR_Block_l1.vi"() -> ("output_Selection_PostR_Block"=w326:i32)  [unwired: 11 in]
      n250 = call "BRig_dataLC_Selection_PostR_Prob_l1.vi"() -> ("output_Selection_PostR_Prob"=w325:i32)  [unwired: 11 in]
      n251 = call "BRig_dataLC_Selection_PostR_Delay_l1.vi"() -> ("output_Selection_PostR_Delay"=w324:i32)  [unwired: 11 in]
      n252 = call "BRig_dataLC_Selection_PostR_Count_l1.vi"() -> ("output_Selection_PostR_Count"=w323:i32)  [unwired: 11 in]
      n253 = call "BRig_dataLC_Selection_PreR_OnOff_l1.vi"() -> ("output_Selection_PreR_OnOff"=w332:i32)  [unwired: 11 in]
      n254 = call "BRig_dataLC_Selection_PreR_Block_l1.vi"() -> ("output_Selection_PreR_Block"=w331:i32)  [unwired: 11 in]
      n255 = call "BRig_dataLC_Selection_PreR_Prob_l1.vi"() -> ("output_Selection_PreR_Prob"=w330:i32)  [unwired: 11 in]
      n256 = call "BRig_dataLC_Selection_PreR_Delay_l1.vi"() -> ("output_Selection_PreR_Delay"=w329:i32)  [unwired: 11 in]
      n257 = call "BRig_dataLC_Selection_PreR_Count_l1.vi"() -> ("output_Selection_PreR_Count"=w328:i32)  [unwired: 11 in]
      n258 = call "BRig_dataLC_Selection_First_OnOff_l1.vi"() -> ("output_Selection_First_OnOff"=w337:i32)  [unwired: 11 in]
      n259 = call "BRig_dataLC_Selection_First_Block_l1.vi"() -> ("output_Selection_First_Block"=w336:i32)  [unwired: 11 in]
      n260 = call "BRig_dataLC_Selection_First_Prob_l1.vi"() -> ("output_Selection_First_Prob"=w335:i32)  [unwired: 11 in]
      n261 = call "BRig_dataLC_Selection_First_Delay_l1.vi"() -> ("output_Selection_First_Delay"=w334:i32)  [unwired: 11 in]
      n262 = call "BRig_dataLC_Selection_First_Count_l1.vi"() -> ("output_Selection_First_Count"=w333:i32)  [unwired: 11 in]
      n263 = call "BRig_dataLC_Reward_OnOff_l1.vi"() -> ("output_Reward_OnOff"=w304:i32)  [unwired: 11 in]
      n264 = call "BRig_dataLC_Reward_Block_l1.vi"() -> ("output_Reward_Block"=w303:i32)  [unwired: 11 in]
      n265 = call "BRig_dataLC_Reward_Trial_l1.vi"() -> ("output_Reward_Trial"=w302:i32)  [unwired: 11 in]
      n266 = call "BRig_dataLC_Reward_Prob_l1.vi"() -> ("output_Reward_Prob"=w301:i32)  [unwired: 11 in]
      n267 = call "BRig_dataLC_Reward_Delay_l1.vi"() -> ("output_Reward_Delay"=w300:i32)  [unwired: 11 in]
      n268 = call "BRig_dataLC_Wrong_OnOff_l1.vi"() -> ("output_Wrong_OnOff"=w299:i32)  [unwired: 11 in]
      n269 = call "BRig_dataLC_Wrong_Block_l1.vi"() -> ("output_Wrong_Block"=w298:i32)  [unwired: 11 in]
      n270 = call "BRig_dataLC_Wrong_Trial_l1.vi"() -> ("output_Wrong_Trial"=w297:i32)  [unwired: 11 in]
      n271 = call "BRig_dataLC_Wrong_Prob_l1.vi"() -> ("output_Wrong_Prob"=w296:i32)  [unwired: 11 in]
      n272 = call "BRig_dataLC_Wrong_Delay_l1.vi"() -> ("output_Wrong_Delay"=w295:i32)  [unwired: 11 in]
      n273 = Index Array(array=w282, index #1=w304, index #2=w303, index #3=w302, index #4=w301, index #5=w300, index #6=w299, index #7=w298, index #8=w297, index #9=w296, index #10=w295) -> (element #1=w292:u16, element #2=w291:u16, element #3=w290:u16, element #4=w289:u16, element #5=w288:u16, element #6=w287:u16, element #7=w286:u16, element #8=w285:u16, element #9=w284:u16, element #10=w283:u16)
      n274 = Index Array(array=w282, index #1=w337, index #2=w336, index #3=w335, index #4=w334, index #5=w333, index #6=w332, index #7=w331, index #8=w330, index #9=w329, index #10=w328, index #11=w327, index #12=w326, index #13=w325, index #14=w324, index #15=w323) -> (element #1=w319:u16, element #2=w318:u16, element #3=w317:u16, element #4=w316:u16, element #5=w315:u16, element #6=w314:u16, element #7=w313:u16, element #8=w312:u16, element #9=w311:u16, element #10=w310:u16, element #11=w309:u16, element #12=w308:u16, element #13=w307:u16, element #14=w306:u16, element #15=w305:u16)
      n275 = Not Equal To 0?(x=w292) -> (x != 0?=w294:bool)
      n276 = Not Equal To 0?(x=w287) -> (x != 0?=w293:bool)
      n277 = Not Equal To 0?(x=w319) -> (x != 0?=w322:bool)
      n278 = Not Equal To 0?(x=w314) -> (x != 0?=w321:bool)
      n279 = Not Equal To 0?(x=w309) -> (x != 0?=w320:bool)
      n280 = local write "LC_Reward_OnOff"(w294) -> ()
      n281 = local write "LC_Reward_Block"(w291) -> ()
      n282 = local write "LC_Reward_Trial"(w290) -> ()
      n283 = local write "LC_Reward_Probability"(w289) -> ()
      n284 = local write "LC_Reward_Tdelay"(w288) -> ()
      n285 = local write "LC_Wrong_OnOff"(w293) -> ()
      n286 = local write "LC_Wrong_Block"(w286) -> ()
      n287 = local write "LC_Wrong_Trial"(w285) -> ()
      n288 = local write "LC_Wrong_Probability"(w284) -> ()
      n289 = local write "LC_Wrong_Tdelay"(w283) -> ()
      n290 = local write "LC_Sel_First_OnOff"(w322) -> ()
      n291 = local write "LC_Sel_First_Block"(w318) -> ()
      n292 = local write "LC_Sel_First_Probability"(w317) -> ()
      n293 = local write "LC_Sel_First_Tdelay"(w316) -> ()
      n294 = local write "LC_Sel_First_Count"(w315) -> ()
      n295 = local write "LC_Sel_PreR_OnOff"(w321) -> ()
      n296 = local write "LC_Sel_PreR_Block"(w313) -> ()
      n297 = local write "LC_Sel_PreR_Probability"(w312) -> ()
      n298 = local write "LC_Sel_PreR_Tdelay"(w311) -> ()
      n299 = local write "LC_Sel_PreR_Count"(w310) -> ()
      n300 = local write "LC_Sel_PostR_OnOff"(w320) -> ()
      n301 = local write "LC_Sel_PostR_Block"(w308) -> ()
      n302 = local write "LC_Sel_PostR_Probability"(w307) -> ()
      n303 = local write "LC_Sel_PostR_Tdelay"(w306) -> ()
      n304 = local write "LC_Sel_PostR_Count"(w305) -> ()
    }
  }
  "output_dataLC" <- w4
  "output_dataExp" <- w1
